vi "test plot t90.vi"() -> ()   [LabVIEW 2019]
panel:
  out "standard error":string
  out "standard output":string
  out "error out":errorcluster
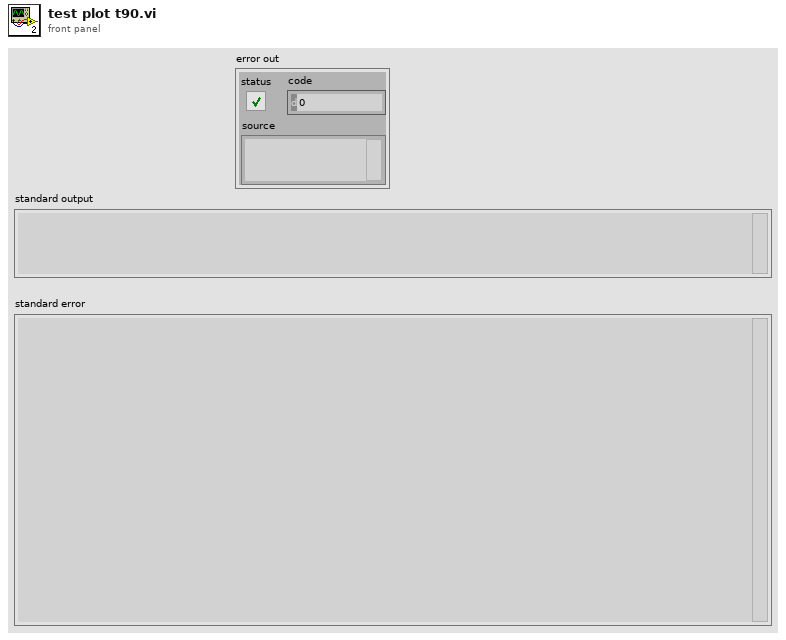
[diagram p1: front panel]
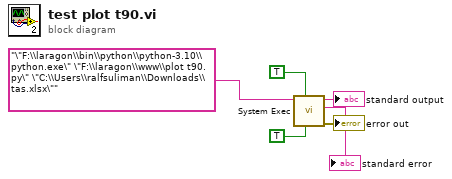
[diagram p0: block diagram]
diagram:
  n1 = call <vilib>:"System Exec.vi"("run minimized? (F)"=TRUE, "wait until completion? (T)"=TRUE, "command line"="\"F:\\laragon\\bin\\python\\python-3.10\\python.exe\" \"F:\\laragon\\www\\plot t90.py\" \"C:\\Users\\ralfsuliman\\Downloads\\tas.xlsx\"") -> ("error out"=→"error out":errorcluster, "standard error"=→"standard error":string, "standard output"=→"standard output":string)  [unwired: 5 in, 1 out]
